vi "WS1050_51 VPI Header_Ver1.4.vi"(0 "VPI Name":string[](array[string])=["All_Drivers OFF", "All Drivers ON", "All Drivers OFF2"], 5 "VPI_Cmd":string[](array[string])=["000000", "3B3B3B", "000000"], 7 "Cmin/Act":bool, 9 "WS1050/51":bool=TRUE, 11 "error in (no error)":errorcluster) -> (4 "VPI Header":string[](array[string]), 6 "VPI_ALL":string[](array[string]), 10 "Cmd_ALL":string[](array[string]), 15 "error out":errorcluster)   [LabVIEW 2012]
panel:
  in  "VPI_Cmd Cmin":string[](array[string])=["000000", "000000", "000000"]
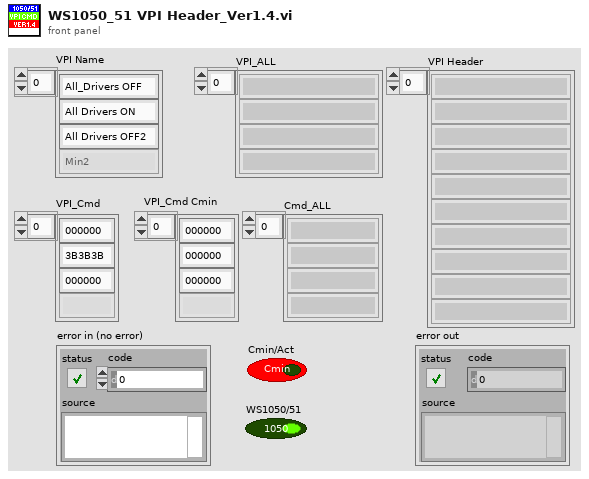
[diagram p1: front panel]
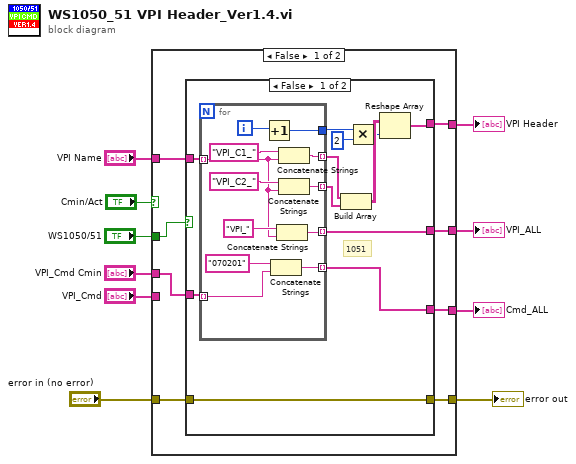
[diagram p0: block diagram]
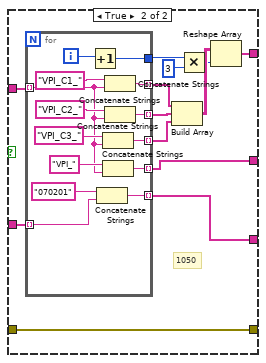
[diagram p2: hidden frame]
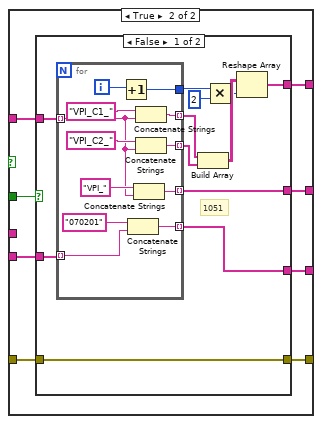
[diagram p3: hidden frame]
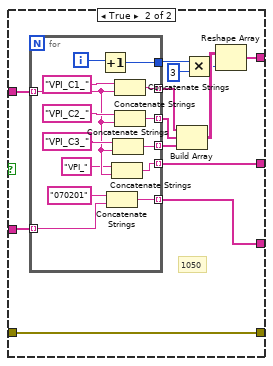
[diagram p4: hidden frame]
diagram:
  n1 = case shown="False" "Cmin/Act" {
    tunnel: "error in (no error)" -> [w13 w77]
    tunnel: [w12 w76] -> w9
    tunnel: "WS1050/51" -> [w14 w75]
    tunnel: "VPI_Cmd" -> [_ w74]
    tunnel: "VPI Name" -> [w15 w73]
    tunnel: [w18 w72] -> w5
    tunnel: [w11 w71] -> w4
    tunnel: [w17 w70] -> w3
    tunnel: "VPI_Cmd Cmin" -> [w16 _]
    frame False {
      n2 = case shown="False" w14 {
        tunnel: [w24 w51] -> w18
        tunnel: [w19 w43] -> w17
        tunnel: w16 -> [w26 w47]
        tunnel: w15 -> [w25 w46]
        tunnel: w13 -> [w21 w45]
        tunnel: [w21 w45] -> w12
        tunnel: [w20 w44] -> w11
        frame False {
          # "1051"
          n3 = for {
            tunnel: w25 -> [w31] mode=indexing
            tunnel: w26 -> [w35] mode=indexing
            tunnel: [w39] -> w23 mode=indexing
            tunnel: [w38] -> w22 mode=indexing
            tunnel: [w37] -> w20 mode=indexing
            tunnel: [w34] -> w19 mode=indexing
            tunnel: [w32] -> w29
            i -> [w33]
            n4 = Increment(x=w33) -> (x+1=w32:i32)
            n5 = Concatenate Strings("070201" ("string"), w35) -> (w34:string)
            n6 = Concatenate Strings("VPI_" ("string"), w31) -> (w37:string)
            n7 = Concatenate Strings("VPI_C1_" ("string"), w31) -> (w39:string)
            n8 = Concatenate Strings("VPI_C2_" ("string"), w31) -> (w38:string)
          }
          n9 = Build Array(w23, w22) -> (w30:string[][])
          n10 = Multiply(x=w29, y=2) -> (x*y=w28:i32)
          n11 = Reshape Array(w30, w28) -> (w24:string[])
        }
        frame True {
          # "1050"
          n12 = for {
            tunnel: w46 -> [w57] mode=indexing
            tunnel: w47 -> [w62] mode=indexing
            tunnel: [w66] -> w50 mode=indexing
            tunnel: [w65] -> w49 mode=indexing
            tunnel: [w64] -> w48 mode=indexing
            tunnel: [w59] -> w43 mode=indexing
            tunnel: [w60] -> w54
            tunnel: [w56] -> w44 mode=indexing
            i -> [w61]
            n13 = Increment(x=w61) -> (x+1=w60:i32)
            n14 = Concatenate Strings("070201" ("string"), w62) -> (w59:string)
            n15 = Concatenate Strings("VPI_C3_" ("string"), w57) -> (w64:string)
            n16 = Concatenate Strings("VPI_" ("string"), w57) -> (w56:string)
            n17 = Concatenate Strings("VPI_C1_" ("string"), w57) -> (w66:string)
            n18 = Concatenate Strings("VPI_C2_" ("string"), w57) -> (w65:string)
          }
          n19 = Build Array(w50, w49, w48) -> (w55:string[][])
          n20 = Multiply(x=w54, y=3) -> (x*y=w53:i32)
          n21 = Reshape Array(w55, w53) -> (w51:string[])
        }
      }
    }
    frame True {
      n22 = case shown="False" w75 {
        tunnel: w77 -> [w80 w110]
        tunnel: [w80 w110] -> w76
        tunnel: w74 -> [w84 w109]
        tunnel: w73 -> [w85 w108]
        tunnel: [w83 w107] -> w72
        tunnel: [w79 w103] -> w71
        tunnel: [w78 w102] -> w70
        frame False {
          # "1051"
          n23 = for {
            tunnel: w85 -> [w90] mode=indexing
            tunnel: w84 -> [w94] mode=indexing
            tunnel: [w98] -> w82 mode=indexing
            tunnel: [w97] -> w81 mode=indexing
            tunnel: [w96] -> w79 mode=indexing
            tunnel: [w93] -> w78 mode=indexing
            tunnel: [w91] -> w88
            i -> [w92]
            n24 = Increment(x=w92) -> (x+1=w91:i32)
            n25 = Concatenate Strings("070201" ("string"), w94) -> (w93:string)
            n26 = Concatenate Strings("VPI_" ("string"), w90) -> (w96:string)
            n27 = Concatenate Strings("VPI_C1_" ("string"), w90) -> (w98:string)
            n28 = Concatenate Strings("VPI_C2_" ("string"), w90) -> (w97:string)
          }
          n29 = Build Array(w82, w81) -> (w89:string[][])
          n30 = Multiply(x=w88, y=2) -> (x*y=w87:i32)
          n31 = Reshape Array(w89, w87) -> (w83:string[])
        }
        frame True {
          # "1050"
          n32 = for {
            tunnel: w108 -> [w117] mode=indexing
            tunnel: w109 -> [w121] mode=indexing
            tunnel: [w125] -> w106 mode=indexing
            tunnel: [w124] -> w105 mode=indexing
            tunnel: [w123] -> w104 mode=indexing
            tunnel: [w118] -> w102 mode=indexing
            tunnel: [w119] -> w113
            tunnel: [w115] -> w103 mode=indexing
            i -> [w120]
            n33 = Increment(x=w120) -> (x+1=w119:i32)
            n34 = Concatenate Strings("070201" ("string"), w121) -> (w118:string)
            n35 = Concatenate Strings("VPI_" ("string"), w117) -> (w115:string)
            n36 = Concatenate Strings("VPI_C3_" ("string"), w117) -> (w123:string)
            n37 = Concatenate Strings("VPI_C1_" ("string"), w117) -> (w125:string)
            n38 = Concatenate Strings("VPI_C2_" ("string"), w117) -> (w124:string)
          }
          n39 = Build Array(w106, w105, w104) -> (w114:string[][])
          n40 = Multiply(x=w113, y=3) -> (x*y=w112:i32)
          n41 = Reshape Array(w114, w112) -> (w107:string[])
        }
      }
    }
  }
  "error out" <- w9
  "VPI_ALL" <- w4
  "Cmd_ALL" <- w3
  "VPI Header" <- w5
